vi "Unit Test 1.vi"   [LabVIEW 2014, in "TableLogger_SQLite_Actor.lvlib" / "TableLogger_SQLite_Actor.lvclass"]
uses:
  TableLogger_SQLite_Actor.lvclass
  TableLogger_Actor/TableLoggerConfig.ctl
  TableLogger_Actor/TableLoggerTypes.ctl
  TableLogger_Actor/TableLogger_Actor.lvlib
types:
  T1 = typedef "TableLogger_Actor.lvlib/TableLoggerConfig.ctl" = cluster{"TableLogger":T2, "DB File Path":path, "DB Backup Interval (Hours)":i32, "Max DB Size (MB)":i32, "Backup Directory":path}
  T2 = typedef "TableLogger_Actor.lvlib/TableLoggerTypes.ctl" = enum16{"CSV Logger", "SQLite Logger"}
  T3 = cluster{"FC Flow Set":dbl, "FM Flow Measure":dbl, "UUT Data":dbl, "Stage 1  Flow Meas":cluster{"FC Flow Set":dbl, "FM Flow Measure":dbl, "UUT Data":dbl}[]}[]
  T4 = cluster{"Test Start Timestamp":timestamp, "Test End Timestamp":timestamp, "Test Jig Location":string, "Location Time Offset":string, "Test Jig ID":string, "Test Jig Fluid":enum16{"DI", "N2"}, "Test Jig Flow":enum16{"Low", "High"}, "Control Board SN":string, "Site Number":i32, "Operator ID":string, "Operation Number":string, "DUT Serial Number":string, "DUT Product Number":string, "DUT Flow Range":i32, "DUT FW Revision":string, "DUT TP1 Offset":dbl, "DUT TP2 Offset":dbl, "DUT Cut Off1":dbl, "DUT Cut Off2":dbl, "PreCal Flow Meas":cluster{"FC Flow Set":dbl, "FM Flow Measure":dbl, "UUT Data":dbl}[], "PostCal Flow Meas":cluster{"FC Flow Set":dbl, "FM Flow Measure":dbl, "UUT Data":dbl}[], "DUT_Coeff":dbl[], "DUT_Flow_Error":dbl[], "Calibration Result":enum16{"Pass", "Fail"}}
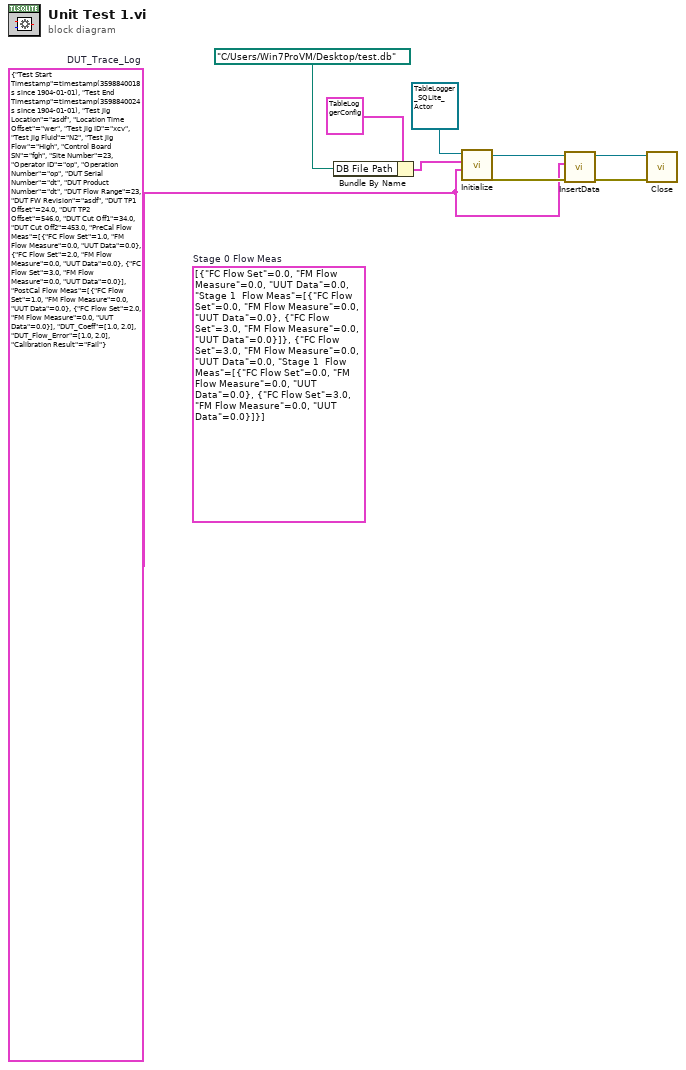
[diagram p0: block diagram]
diagram:
  (unwired) T3 [{"FC Flow Set"=0.0, "FM Flow Measure"=0.0, "UUT Data"=0.0, "Stage 1  Flow Meas"=[{"FC Flow Set"=0.0, "FM Flow Measure"=0.0, "UUT Data"=0.0}, {"FC Flow Set"=3.0, "FM Flow Measure"=0.0, "UUT Data"=0.0}]}, {"FC Flow Set"=3.0, "FM Flow Measure"=0.0, "UUT Data"=0.0, "Stage 1  Flow Meas"=[{"FC Flow Set"=0.0, "FM Flow Measure"=0.0, "UUT Data"=0.0}, {"FC Flow Set"=3.0, "FM Flow Measure"=0.0, "UUT Data"=0.0}]}]  # Stage 0 Flow Meas
  w6 = T4 {"Test Start Timestamp"=timestamp(3598840018.5765285 s since 1904-01-01), "Test End Timestamp"=timestamp(3598840024.2514467 s since 1904-01-01), "Test Jig Location"="asdf", "Location Time Offset"="wer", "Test Jig ID"="xcv", "Test Jig Fluid"=enum."N2", "Test Jig Flow"=enum."High", "Control Board SN"="fgh", "Site Number"=23, "Operator ID"="op", "Operation Number"="op", "DUT Serial Number"="dt", "DUT Product Number"="dt", "DUT Flow Range"=23, "DUT FW Revision"="asdf", "DUT TP1 Offset"=24.0, "DUT TP2 Offset"=546.0, "DUT Cut Off1"=34.0, "DUT Cut Off2"=453.0, "PreCal Flow Meas"=[{"FC Flow Set"=1.0, "FM Flow Measure"=0.0, "UUT Data"=0.0}, {"FC Flow Set"=2.0, "FM Flow Measure"=0.0, "UUT Data"=0.0}, {"FC Flow Set"=3.0, "FM Flow Measure"=0.0, "UUT Data"=0.0}], "PostCal Flow Meas"=[{"FC Flow Set"=1.0, "FM Flow Measure"=0.0, "UUT Data"=0.0}, {"FC Flow Set"=2.0, "FM Flow Measure"=0.0, "UUT Data"=0.0}], "DUT_Coeff"=[1.0, 2.0], "DUT_Flow_Error"=[1.0, 2.0], "Calibration Result"=enum."Fail"}  # DUT_Trace_Log
  n1 = Bundle By Name(cluster=T1 {"TableLogger"=enum."CSV Logger", "DB File Path"=path "", "DB Backup Interval (Hours)"=0, "Max DB Size (MB)"=0, "Backup Directory"=path ""} ("TableLogger Config"), "DB File Path"=path "C:/Users/Win7ProVM/Desktop/test.db" ("DB Path")) -> (w2:T1)
  n2 = call-dynamic "Initialize.vi"("Data Cluster (for Table Headers)"=w6, "TableLogger Config"=w2, "object in"=refnum<class "TableLogger_SQLite_Actor.lvclass"> refnum) -> ("error out"=w7:errorcluster, "object out"=w8:refnum<class "TableLogger_SQLite_Actor.lvclass">)  [unwired: 7 in]
  n3 = call-dynamic "InsertData.vi"("error in (no error)"=w7, "Data Cluster"=w6, "object in"=w8) -> ("error out"=w4:errorcluster, "object out"=w5:refnum<class "TableLogger_SQLite_Actor.lvclass">)  [unwired: 7 in]
  n4 = call-dynamic "Close.vi"("error in (no error)"=w4, "object in"=w5) -> ()  [unwired: 8 in, 2 out]
